vi "LVClass_WavefrontCorrectorSet Read AllValueSetAndGet.vi"(8 "error in (no error)":errorcluster, 11 "WavefrontCorrectorSet in":refnum<class "WavefrontCorrectorSet.lvclass">) -> (0 "error out":errorcluster, 2 "AllValueSetAndGet":T1[](array[typedef]), 3 "WavefrontCorrectorSet out":refnum<class "WavefrontCorrectorSet.lvclass">)   [LabVIEW 2020, in "WavefrontCorrectorSet.lvclass"]
uses:
  WavefrontCorrectorSet.lvclass
  Controls/CameraParametersSetup.ctl
  Controls/CameraParameters_Type.ctl
  WavefrontCorrectorSet.lvclass/WavefrontCorrectorSet.ctl
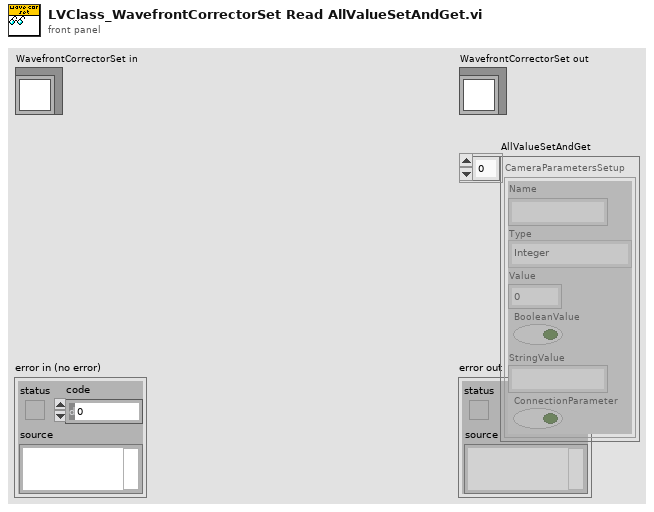
[diagram p1: front panel]
types:
  T1 = typedef "CameraParametersSetup.ctl" = cluster{"Name":string, "Type":T2, "Value":dbl, "BooleanValue":bool, "StringValue":string, "ConnectionParameter":bool}
  T2 = typedef "CameraParameters_Type.ctl" = enum16{"Integer", "Real", "String", "Boolean"}
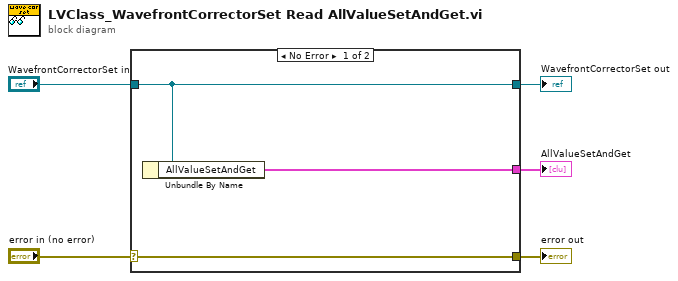
[diagram p0: block diagram]
diagram:
  n1 = case shown="No Error" "error in (no error)" {
    selector: "error in (no error)" -> [w8 w9]
    tunnel: [w8 w9] -> w4
    tunnel: [w7 w10] -> w2
    tunnel: "WavefrontCorrectorSet in" -> [w7 w10]
    tunnel: [w6 _] -> w1
    frame No Error {
      n2 = Unbundle By Name(w7) -> ("AllValueSetAndGet"=w6:T1[])
    }
    frame Error {
    }
  }
  "error out" <- w4
  "WavefrontCorrectorSet out" <- w2
  "AllValueSetAndGet" <- w1
